vi "Container to Index.vi"(10 "Container":T1) -> (2 "Index":i32)   [LabVIEW 2015, in "cRIO-Carbondioxide.lvlib" / "CO2-Actor.lvlib" / "Storage Line.lvclass"]
uses:
  Storage Line.lvclass
  Controls/Sample Transfer Container Enumerator.ctl
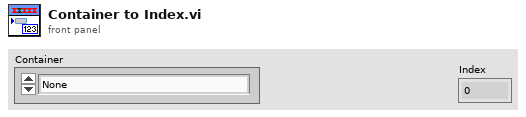
[diagram p1: front panel]
types:
  T1 = typedef "Sample Transfer Container Enumerator.ctl" = enum16{"None", "Sample 1", "Sample 2", "Sample 3", "Sample 4", "Sample 5", "Storage 01", "Storage 02", "Storage 03", "Storage 04", "Storage 05", "Storage 06", "Storage 07", "Storage 08", "Storage 09", "Storage 10", "Storage 11", "Storage 12", "Syringe", "Undefined"}
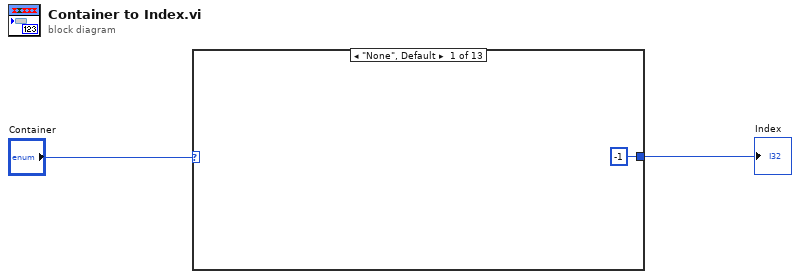
[diagram p0: block diagram]
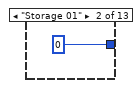
[diagram p2: hidden frame]
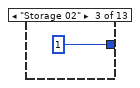
[diagram p3: hidden frame]
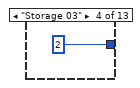
[diagram p4: hidden frame]
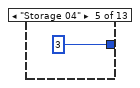
[diagram p5: hidden frame]
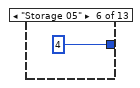
[diagram p6: hidden frame]
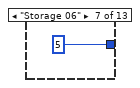
[diagram p7: hidden frame]
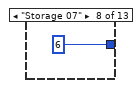
[diagram p8: hidden frame]
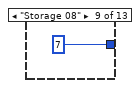
[diagram p9: hidden frame]
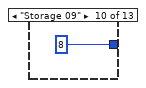
[diagram p10: hidden frame]
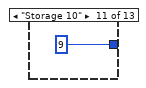
[diagram p11: hidden frame]
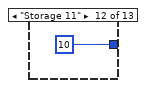
[diagram p12: hidden frame]
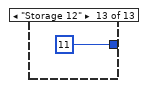
[diagram p13: hidden frame]
diagram:
  n1 = case shown="\"None\", Default" "Container" {
    tunnel: [-1 0 1 2 3 4 5 6 7 8 9 10 11] -> w1
    frame "None", Default {
    }
    frame "Storage 01" {
    }
    frame "Storage 02" {
    }
    frame "Storage 03" {
    }
    frame "Storage 04" {
    }
    frame "Storage 05" {
    }
    frame "Storage 06" {
    }
    frame "Storage 07" {
    }
    frame "Storage 08" {
    }
    frame "Storage 09" {
    }
    frame "Storage 10" {
    }
    frame "Storage 11" {
    }
    frame "Storage 12" {
    }
  }
  "Index" <- w1
